vi "Botones_intensidad_manual.vi"(2 "Seleción método":bool, 8 "Nombre del archivo":string, 9 "Angulo de los elementos opticos":dbl[](array[numeric]), 10 "Directorio scripts matlab 2":path=path "C:/Users/franjas/Documents/rutinas-calibracion-slm", 11 "Run":bool) -> (3 "?":bool)   [LabVIEW 2013]
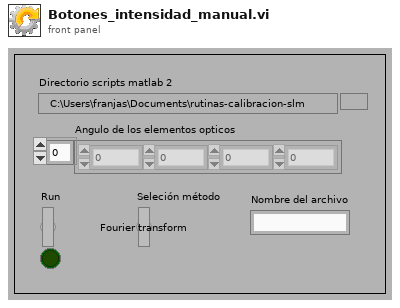
[diagram p1: front panel]
types:
  T1 = enum16{"Escritura", "Med fas", "Conf fase", "Med ampl", "Conf final", "finalizar"}
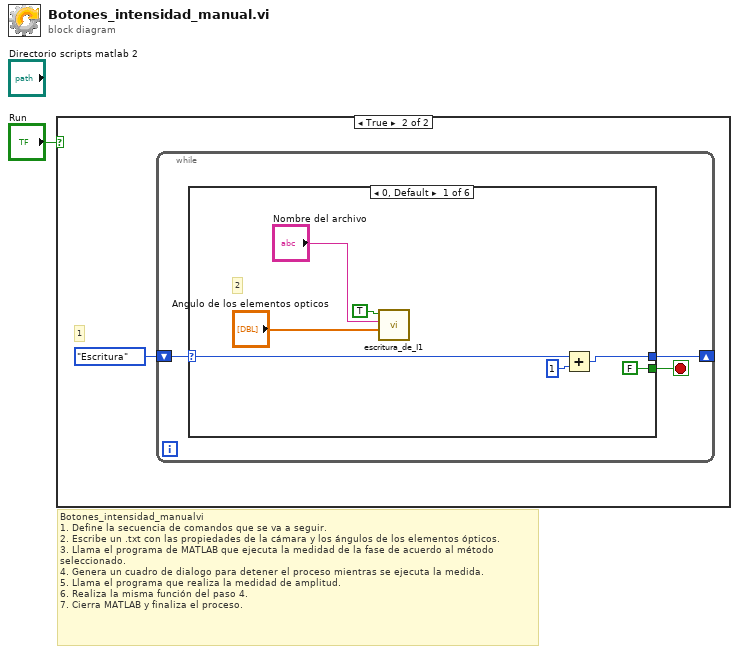
[diagram p0: block diagram]
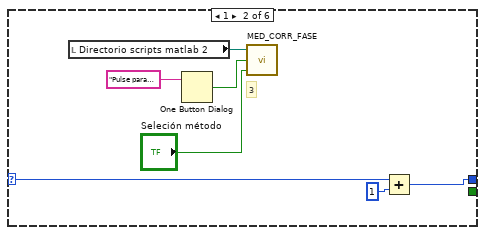
[diagram p3: hidden frame]
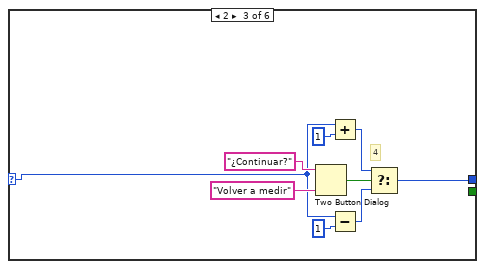
[diagram p4: hidden frame]
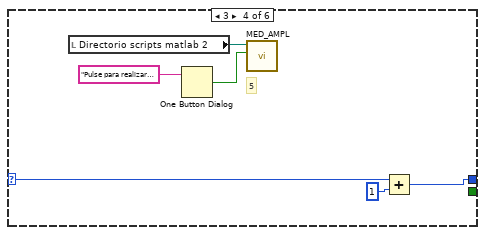
[diagram p5: hidden frame]
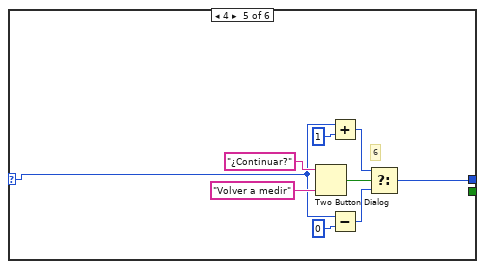
[diagram p6: hidden frame]
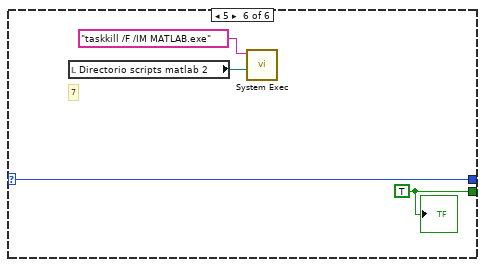
[diagram p7: hidden frame]
diagram:
  # "Botones_intensidad_manualvi\n1. Define la secuencia de comandos que se va a seguir.\n2. Escribe un .txt con las propiedades de la cámara y los ángulos de los elementos ópticos.\n3. Llama el programa de MATLAB que ejecuta la medidad de la fase de acuerdo al método \nseleccionado. \n4. Genera un cuadro de dialogo para detener el proceso mientras se ejecuta la medida.\n5. Llama el programa que realiza la medidad de amplitud.\n6. Realiza la misma función del paso 4.\n7. Cierra MATLAB y finaliza el proceso."
  n1 = case shown="True" "Run" {
    frame False {
    }
    frame True {
      # "1"
      n2 = while {
        shift-right: [w4] -> _
        shift-left: T1."Escritura" -> [w5]
        stop <- w3 stop-if-true
        n3 = case shown="0, Default" w5 {
          selector: w5 -> [w11 w17 w21 w32 w36 w46]
          tunnel: [w12 w16 w23 w31 w38 w46] -> w4
          tunnel: [FALSE ("I1\n<0,0|0,0>") _ _ _ _ w47] -> w3
          frame 0, Default {
            # "2"
            n4 = call "escritura_de_I1.vi"("I1\n<0,0|0,0>"=TRUE ("I1\n<0,0|0,0>"), "String"="Nombre del archivo", "Array"="Angulo de los elementos opticos") -> ()  [unwired: 8 in]
            n5 = Add(x=w11, y=1) -> (x+y=w12:i32)
          }
          frame 1 {
            # "3"
            n6 = local read "Directorio scripts matlab 2"() -> (w14:path)
            n7 = One Button Dialog(message="Pulse para realizar medida de diferencia de fase") -> (true=w15:bool)  [unwired: 1 in]
            n8 = call "MED_CORR_FASE.vi"("Seleción método"="Seleción método", "Ejecucion"=w15, "Directorio scripts matlab"=w14) -> ()
            n9 = Add(x=w17, y=1) -> (x+y=w16:i32)
          }
          frame 2 {
            # "4"
            n10 = Two Button Dialog(message="¿Continuar?", 1:"Volver a medir" ("F button name (\"Cancel\")")) -> (T button?=w26:bool)  [unwired: 1 in]
            n11 = Add(x=w21, y=1) -> (x+y=w20:i32)
            n12 = Subtract(x=w21, y=1) -> (x-y=w24:i32)
            n13 = Select(t=w20, s=w26, f=w24) -> (s? t:f=w23:i32)
          }
          frame 3 {
            # "5"
            n14 = local read "Directorio scripts matlab 2"() -> (w29:path)
            n15 = One Button Dialog(message="Pulse para realizar medidas de amplitud:") -> (true=w30:bool)  [unwired: 1 in]
            n16 = call "MED_AMPL.vi"("Boolean"=w30, "Directorio scripts matlab"=w29) -> ()  [unwired: 10 in]
            n17 = Add(x=w32, y=1) -> (x+y=w31:i32)
          }
          frame 4 {
            # "6"
            n18 = Two Button Dialog(message="¿Continuar?", 1:"Volver a medir" ("F button name (\"Cancel\")")) -> (T button?=w41:bool)  [unwired: 1 in]
            n19 = Add(x=w36, y=1) -> (x+y=w35:i32)
            n20 = Subtract(x=w36, y=0) -> (x-y=w39:i32)
            n21 = Select(t=w35, s=w41, f=w39) -> (s? t:f=w38:i32)
          }
          frame 5 {
            w47 = TRUE
            # "7"
            n22 = local read "Directorio scripts matlab 2"() -> (w45:path)
            n23 = call <vilib>:"System Exec.vi"("working directory"=w45, "command line"="taskkill /F /IM MATLAB.exe") -> ()  [unwired: 6 in, 4 out]
            "?" <- w47
          }
        }
      }
    }
  }
